vi "Doe_Julabo_Control_subVI.vi"(0 "Julabo CF41 VISA":refnum<visa-resource-name>="COM3", 1 "Data Cluster In":T1={"Current DoE"=[], "SSI 1 Flow Rate"=0.0, "SSI 2 Flow Rate"=0.0, "FLOM 1 Flow Rate"=0.0, "FLOM 2 Flow Rate"=0.0, "Pumps Running?"=FALSE, "Boolean 2"=FALSE, "Boolean 3"=FALSE, "Boolean 4"=FALSE, "At Equilibrium?"=FALSE, "Script Running?"=FALSE, "Current Script Iteration"=0.0, "Total Script Iterations"=0.0, "FLOM Pumps VISA"="COM2", "SSI 1 Pump VISA"="COM76", "SSI 2 Pump VISA"="COM74", "Huber Unistat VISA"="COM1", "SSI 3 Pump VISA"="COM76", "SSI 4 Pump VISA"="COM76", "SSI 4 Flow Rate"=0.0, "SSI 3 Flow Rate"=0.0, "Flow Meter 1 Rate "=0.0, "Flow Meter 2 Rate"=0.0, "Flow Meter 3 Rate"=0.0, "Flow Meter 4 Rate"=0.0, "SSI 1 Flow Setpoint"=0.0, "SSI 2 Flow Setpoint"=0.0, "SSI 3 Flow Setpoint"=0.0, "SSI 4 Flow Setpoint"=0.0, "Temperature Setpoint"=0.0, "Flow meter 3 COM"=17, "Flow meter 5 COM"=18, "Flow meter 4 COM"=19, "Flow meter 2 COM"=16, "Flow meter 1 COM"=15, "Unit"=enum."PSI", "Pressure COM"="COM6", "Julabo Setpoint"=0.0, "Julabo Control"=enum."Internal", "Overtemp"=50.0, "Subtemp"=-20.0, "HeatMax"=50, "CoolMax"=-100, "InternMax"=50.0, "InternMin"=0.0, "Upper Bandlimit"=100.0, "Lower Bandlimit"=0.0, "Julabo CF41 VISA"="COM3", "Xp (0.6K) Int"=0.6, "Tn (3s) Int"=3, "Tv (0s) Int"=0, "Dynamic (0: aperiodic) Int"=enum."aperiodic", "Xp (0.6K) Ext"=0.6, "Tn (3s) Ext"=3, "Tv (0s) Ext"=0, "XpU (0.6K) Ext"=0.6} {"XpU (0.6K) Ext" min=0.1 max=99.9; "Tv (0s) Ext" max=999; "Tn (3s) Ext" min=3 max=9999; "Xp (0.6K) Ext" min=0.1 max=99.9; "Tv (0s) Int" max=999; "Tn (3s) Int" min=3 max=9999; "Xp (0.6K) Int" min=0.1 max=99.9; "Lower Bandlimit" min=0.0 max=200.0; "Upper Bandlimit" min=0.0 max=200.0; "InternMin" format="%.2f"; "InternMax" format="%.2f"; "CoolMax" min=-100 max=0; "HeatMax" max=100; "Subtemp" format="%.2f"; "Overtemp" format="%.2f"; "Julabo Setpoint" format="%.2f"; "Current DoE" format="%0.3f"}, 2 "Selector":i32, 5 "Serial Configuration":T4={"Baud Rate"=4800, "Parity"=2, "Data Bits"=7, "Stop Bits"=10, "Flow Control"=2} {"Flow Control" items=["None", "XON/XOFF", "RTS/CTS", "XON/XOFF & RTS/CTS", "DTR/DSR", "XON/XOFF & DTR/DSR"]; "Stop Bits" items=["1.0"=10, "1.5"=15, "2.0"=20]; "Data Bits" items=["7"=7, "8"=8]; "Parity" items=["None", "Odd", "Even", "Mark", "Space"]; "Baud Rate" items=["300"=300, "600"=600, "1200"=1200, "2400"=2400, "4800"=4800, "9600"=9600, "19200"=19200]}, 7 "RS485-Address (128: RS232)":u32=128, 9 "ID Query? (T: Yes)":bool=TRUE) -> (4 "Data Cluster Out":T1={"Current DoE"=[], "SSI 1 Flow Rate"=0.0, "SSI 2 Flow Rate"=0.0, "FLOM 1 Flow Rate"=0.0, "FLOM 2 Flow Rate"=0.0, "Pumps Running?"=FALSE, "Boolean 2"=FALSE, "Boolean 3"=FALSE, "Boolean 4"=FALSE, "At Equilibrium?"=FALSE, "Script Running?"=FALSE, "Current Script Iteration"=0.0, "Total Script Iterations"=0.0, "FLOM Pumps VISA"="COM2", "SSI 1 Pump VISA"="COM76", "SSI 2 Pump VISA"="COM74", "Huber Unistat VISA"="COM1", "SSI 3 Pump VISA"="COM76", "SSI 4 Pump VISA"="COM76", "SSI 4 Flow Rate"=0.0, "SSI 3 Flow Rate"=0.0, "Flow Meter 1 Rate "=0.0, "Flow Meter 2 Rate"=0.0, "Flow Meter 3 Rate"=0.0, "Flow Meter 4 Rate"=0.0, "SSI 1 Flow Setpoint"=0.0, "SSI 2 Flow Setpoint"=0.0, "SSI 3 Flow Setpoint"=0.0, "SSI 4 Flow Setpoint"=0.0, "Temperature Setpoint"=0.0, "Flow meter 3 COM"=17, "Flow meter 5 COM"=18, "Flow meter 4 COM"=19, "Flow meter 2 COM"=16, "Flow meter 1 COM"=15, "Unit"=enum."PSI", "Pressure COM"="COM6", "Julabo Setpoint"=0.0, "Julabo Control"=enum."Internal", "Overtemp"=50.0, "Subtemp"=-20.0, "HeatMax"=50, "CoolMax"=-100, "InternMax"=50.0, "InternMin"=0.0, "Upper Bandlimit"=100.0, "Lower Bandlimit"=0.0, "Julabo CF41 VISA"="COM3", "Xp (0.6K) Int"=0.6, "Tn (3s) Int"=3, "Tv (0s) Int"=0, "Dynamic (0: aperiodic) Int"=enum."aperiodic", "Xp (0.6K) Ext"=0.6, "Tn (3s) Ext"=3, "Tv (0s) Ext"=0, "XpU (0.6K) Ext"=0.6} {"XpU (0.6K) Ext" min=0.1 max=99.9; "Tv (0s) Ext" max=999; "Tn (3s) Ext" min=3 max=9999; "Xp (0.6K) Ext" min=0.1 max=99.9; "Tv (0s) Int" max=999; "Tn (3s) Int" min=3 max=9999; "Xp (0.6K) Int" min=0.1 max=99.9; "Lower Bandlimit" min=0.0 max=200.0; "Upper Bandlimit" min=0.0 max=200.0; "InternMin" format="%.2f"; "InternMax" format="%.2f"; "CoolMax" min=-100 max=0; "HeatMax" max=100; "Subtemp" format="%.2f"; "Overtemp" format="%.2f"; "Julabo Setpoint" format="%.2f"; "Current DoE" format="%0.3f"}, 15 "device error out":errorcluster)   [LabVIEW 2015, in "JULABO DeviceDriver.lvlib"]
doc: "Advanced event triggered example"
uses:
  <instrlib>/JULABO DeviceDriver/JULABO DeviceDriver.lvlib
  <instrlib>/JULABO DeviceDriver/Examples/Julabo Serial Control.ctl
  --Controls and TypeDefs--/DoE_Control_Cluster.ctl
panel:
  in  "Xp (0.6K) 2":dbl=0.6 min=0.1 max=99.9
  in  "Tn (3s) 2":u16=3 min=3 max=9999
  in  "Tv (0s) 2":u16 max=999
  in  "XpU (0.6K)":dbl=0.6 min=0.1 max=99.9
  in  "Xp (0.6K)":dbl=0.6 min=0.1 max=99.9
  in  "Tn (3s)":u16=3 min=3 max=9999
  in  "Tv (0s)":u16 max=999
  in  "Dynamic (0: aperiodic)":enum16{"aperiodic", "standard"}(ring)
  in  "Control":enum16{"Internal", "External"}(ring)
  out "Internal Temp":dbl format="%.2f"
  out "External Temp":dbl format="%.2f"
  out "Safety Temp":dbl
  out "Excess Temp Protection":dbl
  in  "Setpoint":dbl format="%.2f"
  in  "StartStop":bool
  in  "Upper Bandlimit":dbl=100.0 min=0.0 max=200.0
  in  "Lower Bandlimit":dbl min=0.0 max=200.0
  in  "InternMax":dbl=50.0 format="%.2f"
  in  "InternMin":dbl format="%.2f"
  in  "HeatMax":u8=50 max=100
  in  "CoolMax":i8=-100 min=-100 max=0
  in  "Overtemp":dbl=50.0 format="%.2f"
  in  "Subtemp":dbl=-20.0 format="%.2f"
  out "error out 2":errorcluster caption="error out"
  out "error out":errorcluster
  in  "Registerkartenelement":T2(tab)
  out "Power":i8(slide) scale=-100.0..100.0
  out "Diagram":T3(graph)
  in  "Stopp":bool
  in  "Reset / Default (T: Both)":bool=TRUE
  # "Note: Julabo must be set to Set Temp - RS232\nfor commands to properly write to unit!!!!!"
  # "1. Select the COM-Port and adjust the serial\nconfiguration for your instrument\n2. Adjust the Read cycle\n3. Start the VI by pressing the \"Start\" -Button\n( Arrow button on the top-left corner)\n4. To stop the execution press the \"Stop\" button"
  # "Julabo"
  # "Limits"
  # "PID Control Parameters"
  # "Julabo"
  # "Limits"
  # "PID Control Parameters"
  # "Internal parameters"
  # "External parameters"
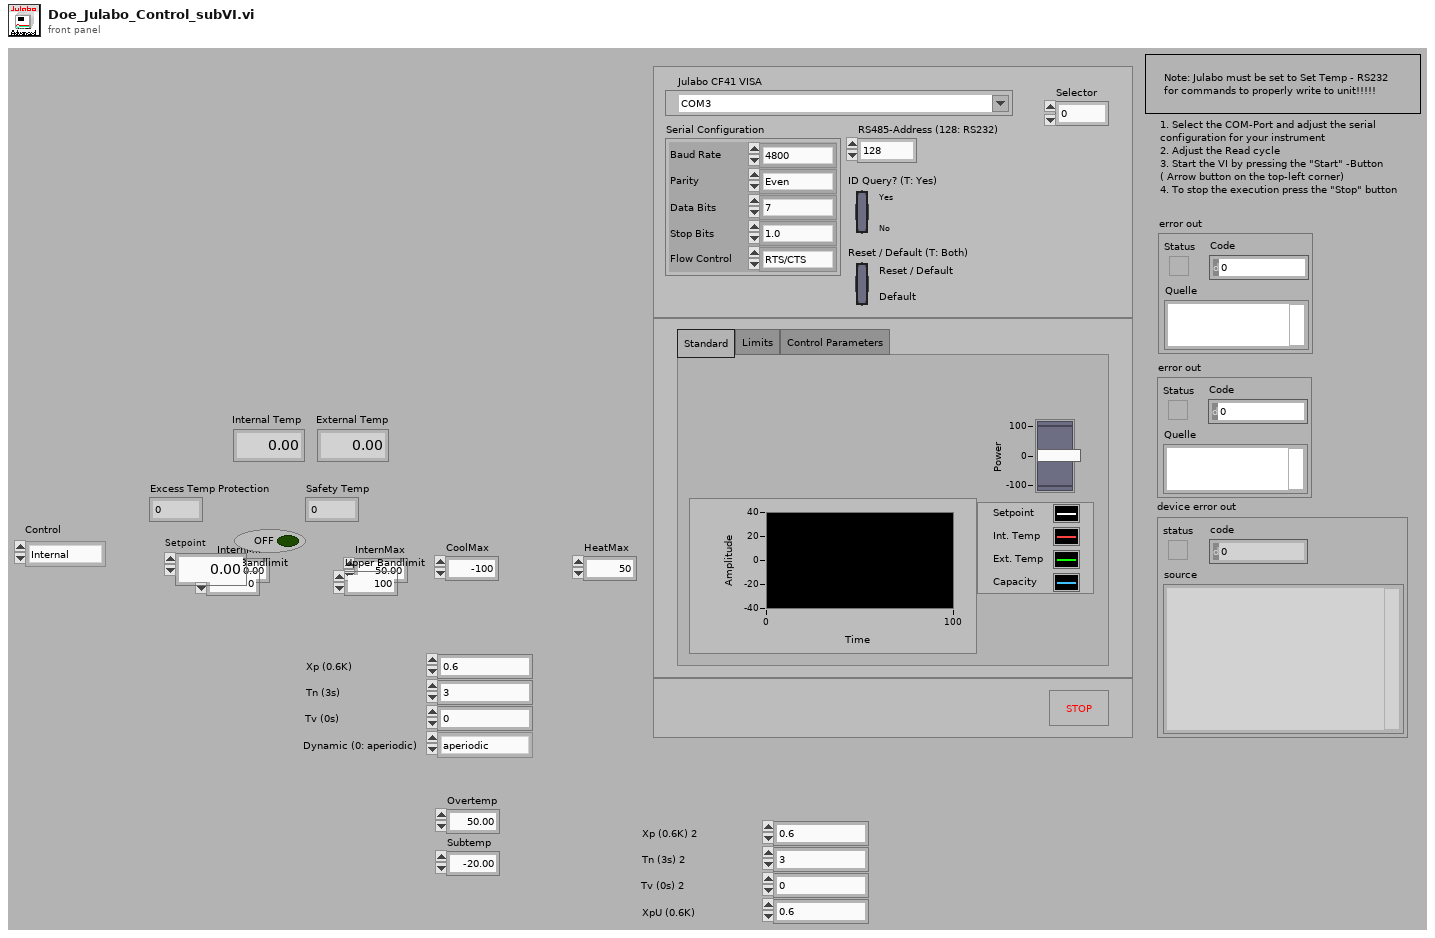
[diagram p1: front panel]
types:
  T1 = typedef "DoE_Control_Cluster.ctl" = cluster{"Current DoE":dbl[][], "SSI 1 Flow Rate":dbl, "SSI 2 Flow Rate":dbl, "FLOM 1 Flow Rate":dbl, "FLOM 2 Flow Rate":dbl, "Pumps Running?":bool, "Boolean 2":bool, "Boolean 3":bool, "Boolean 4":bool, "At Equilibrium?":bool, "Script Running?":bool, "Current Script Iteration":dbl, "Total Script Iterations":dbl, "FLOM Pumps VISA":refnum<visa-resource-name>, "SSI 1 Pump VISA":refnum<visa-resource-name>, "SSI 2 Pump VISA":refnum<visa-resource-name>, "Huber Unistat VISA":refnum<visa-resource-name>, "SSI 3 Pump VISA":refnum<visa-resource-name>, "SSI 4 Pump VISA":refnum<visa-resource-name>, "SSI 4 Flow Rate":dbl, "SSI 3 Flow Rate":dbl, "Flow Meter 1 Rate ":dbl, "Flow Meter 2 Rate":dbl, "Flow Meter 3 Rate":dbl, "Flow Meter 4 Rate":dbl, "SSI 1 Flow Setpoint":dbl, "SSI 2 Flow Setpoint":dbl, "SSI 3 Flow Setpoint":dbl, "SSI 4 Flow Setpoint":dbl, "Temperature Setpoint":dbl, "Flow meter 3 COM":u16, "Flow meter 5 COM":u16, "Flow meter 4 COM":u16, "Flow meter 2 COM":u16, "Flow meter 1 COM":u16, "Unit":enum16{"PSI", "Bar", "cm H2O", "ft H2O", "hectoPascal", "in Hg", "in H2O", "kiloPascal", "milliBar", "mmHg", "MegaPascal", "Numeric Pressure"}, "Pressure COM":refnum<visa-resource-name>, "Julabo Setpoint":dbl, "Julabo Control":enum16{"Internal", "External"}, "Overtemp":dbl, "Subtemp":dbl, "HeatMax":u8, "CoolMax":i8, "InternMax":dbl, "InternMin":dbl, "Upper Bandlimit":dbl, "Lower Bandlimit":dbl, "Julabo CF41 VISA":refnum<visa-resource-name>, "Xp (0.6K) Int":dbl, "Tn (3s) Int":u16, "Tv (0s) Int":u16, "Dynamic (0: aperiodic) Int":enum16{"aperiodic", "standard"}, "Xp (0.6K) Ext":dbl, "Tn (3s) Ext":u16, "Tv (0s) Ext":u16, "XpU (0.6K) Ext":dbl}
  T2 = enum32{"Standard", "Limits", "Control Parameters"}
  T3 = cluster{"Setpoint (out)":dbl, "InternalTemp (out)":dbl, "ExternalTemp (out)":dbl, "Capacity (out)":i8}
  T4 = typedef "Julabo Serial Control.ctl" = cluster{"Baud Rate":u32, "Parity":u16, "Data Bits":u16, "Stop Bits":u16, "Flow Control":u16}
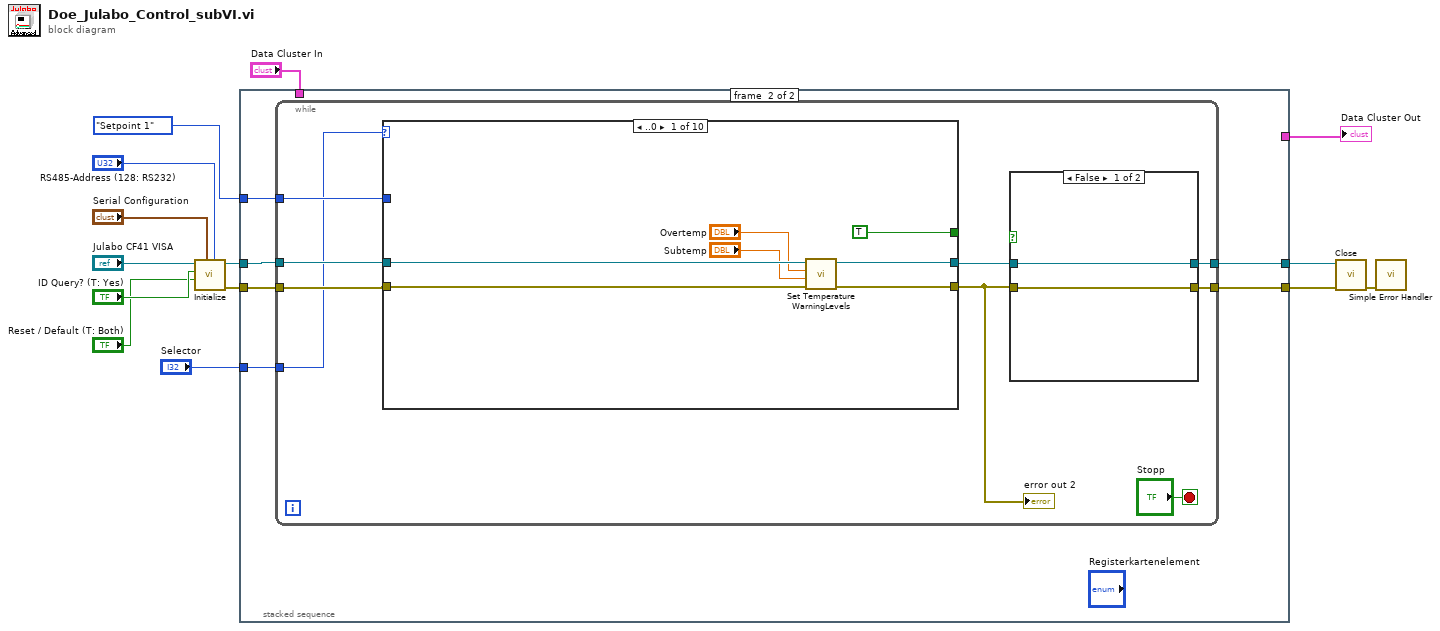
[diagram p0: block diagram]
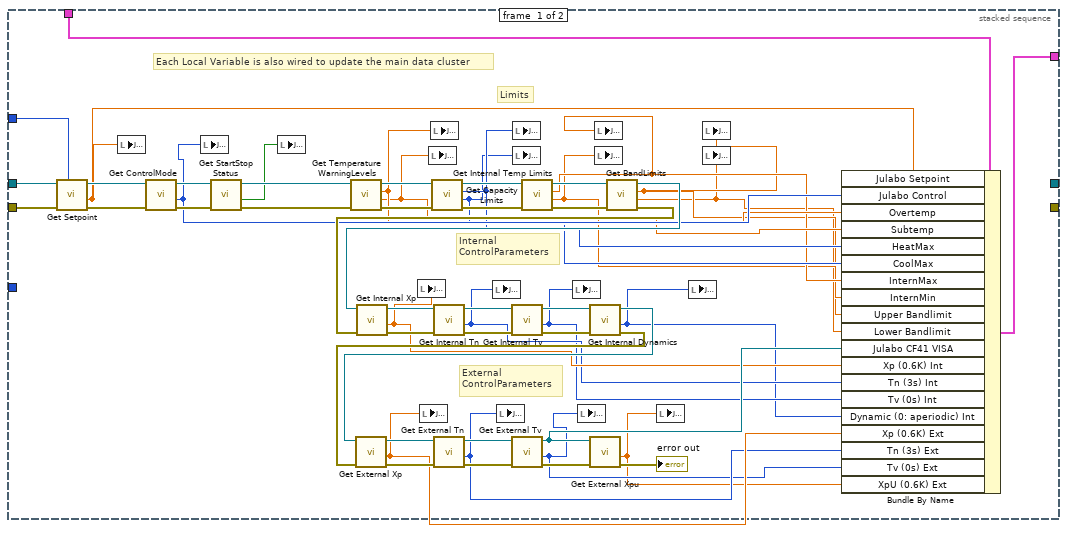
[diagram p2: hidden frame]
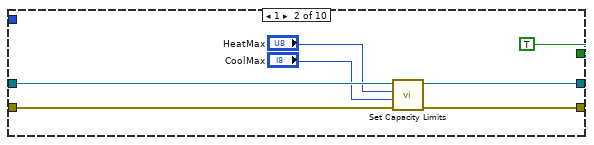
[diagram p3: hidden frame]
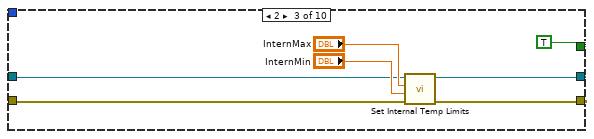
[diagram p4: hidden frame]
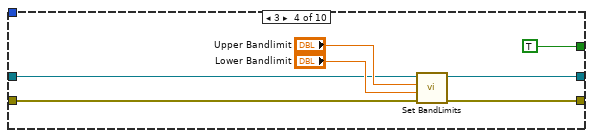
[diagram p5: hidden frame]
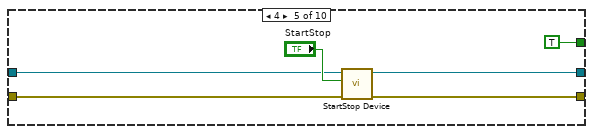
[diagram p6: hidden frame]
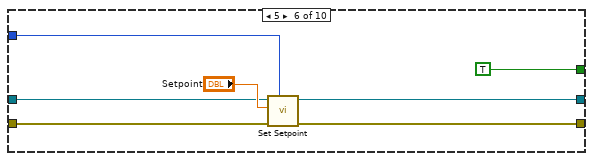
[diagram p7: hidden frame]
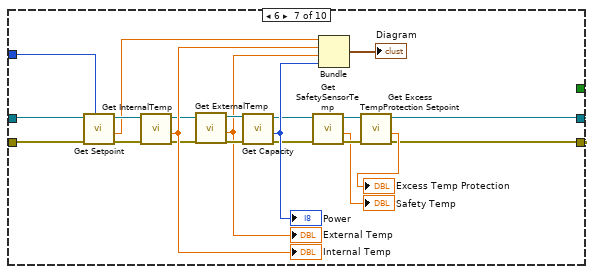
[diagram p8: hidden frame]
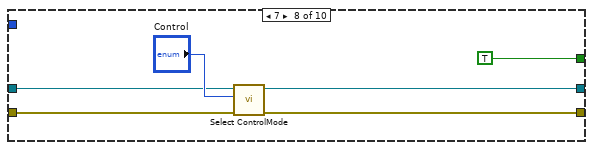
[diagram p9: hidden frame]
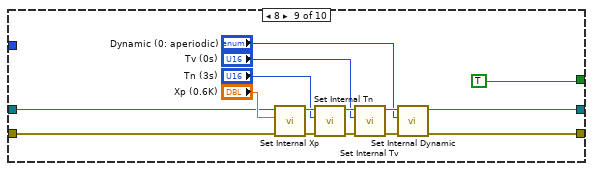
[diagram p10: hidden frame]
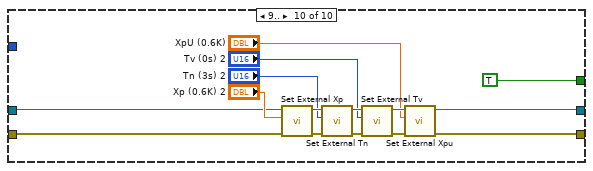
[diagram p11: hidden frame]
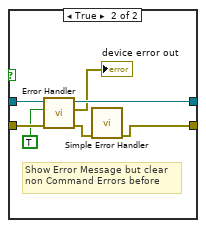
[diagram p12: hidden frame]
diagram:
  n1 = call <instrlib>:"Initialize.vi"("RS485-Address (128: RS232)"="RS485-Address (128: RS232)", "Serial Configuration"="Serial Configuration", "Reset / Default (T: Both)"="Reset / Default (T: Both)", "ID Query? (T: Yes)"="ID Query? (T: Yes)", "VISA resource name"="Julabo CF41 VISA") -> ("error out"=w7:errorcluster, "VISA resource name out"=w8:refnum<visa-resource-name>)  [unwired: 5 in]
  n2 = stacked-sequence {
    tunnel: w8 -> [w40 w69]
    tunnel: w7 -> [w39 w70]
    tunnel: [_ w73] -> w6
    tunnel: [_ w72] -> w5
    tunnel: enum16{"Setpoint 1", "Setpoint 2", "Setpoint 3"}."Setpoint 1" ("Setpointindex") -> [w36 w71]
    tunnel: "Data Cluster In" -> [w35 _]
    tunnel: [w34 _] -> w2
    tunnel: "Selector" -> [_ w68]
    frame #0 {
      # "Each Local Variable is also wired to update the main data cluster"
      # "External\nControlParameters"
      # "Internal\nControlParameters"
      # "Limits"
      n3 = call <instrlib>:"Get Setpoint.vi"("Setpointindex"=w36, "error in (no error)"=w39, "VISA resource name"=w40) -> ("error out"=w37:errorcluster, "Setpoint (out)"=w33:dbl, "VISA resource name out"=w38:refnum<visa-resource-name>)  [unwired: 6 in]
      n4 = local write item#-1(w33) -> ()
      n5 = call <instrlib>:"Get ControlMode.vi"("error in"=w37, "VISA resource name in"=w38) -> ("error out"=w42:errorcluster, "Control (out)"=w32:enum16{"Internal", "External"}, "VISA resource name out"=w46:refnum<visa-resource-name>)  [unwired: 7 in]
      n6 = local write item#-1(w32) -> ()
      n7 = call <instrlib>:"Get StartStop Status.vi"("error in"=w42, "VISA resource name in"=w46) -> ("error out"=w41:errorcluster, "Status"=w43:bool, "VISA resource name out"=w44:refnum<visa-resource-name>)  [unwired: 7 in]
      n8 = local write item#-1(w43) -> ()
      n9 = call <instrlib>:"Get Temperature WarningLevels.vi"("error in (no error)"=w41, "VISA resource name"=w44) -> ("error out"=w64:errorcluster, "Subtemp (out)"=w30:dbl, "Overtemp (out)"=w31:dbl, "VISA resource name out"=w67:refnum<visa-resource-name>)  [unwired: 2 in]
      n10 = local write item#-1(w30) -> ()
      n11 = local write item#-1(w31) -> ()
      n12 = call <instrlib>:"Get Capacity Limits.vi"("error in (no error)"=w64, "VISA resource name"=w67) -> ("error out"=w63:errorcluster, "Maximum cooling capacity(out)"=w28:i8, "Maximum heating capacity(out)"=w29:u8, "VISA resource name out"=w66:refnum<visa-resource-name>)  [unwired: 2 in]
      n13 = local write item#-1(w29) -> ()
      n14 = local write item#-1(w28) -> ()
      n15 = call <instrlib>:"Get Internal Temp Limits.vi"("error in (no error)"=w63, "VISA resource name"=w66) -> ("error out"=w62:errorcluster, "IntMin (out)"=w26:dbl, "IntMax (out)"=w27:dbl, "VISA resource name out"=w65:refnum<visa-resource-name>)  [unwired: 2 in]
      n16 = local write item#-1(w27) -> ()
      n17 = local write item#-1(w26) -> ()
      n18 = call <instrlib>:"Get BandLimits.vi"("error in (no error)"=w62, "VISA resource name"=w65) -> ("error out"=w54:errorcluster, "LowerBand (out)"=w24:dbl, "UpperBand (out)"=w25:dbl, "VISA resource name out"=w55:refnum<visa-resource-name>)  [unwired: 2 in]
      n19 = call <instrlib>:"Get Internal Xp.vi"("error in"=w54, "VISA resource name in"=w55) -> ("error out"=w56:errorcluster, "InternalXp (out)"=w22:dbl, "VISA resource name out"=w57:refnum<visa-resource-name>)  [unwired: 7 in]
      n20 = local write item#-1(w22) -> ()
      n21 = call <instrlib>:"Get Internal Tn.vi"("error in"=w56, "VISA resource name in"=w57) -> ("error out"=w58:errorcluster, "InternalTn (out)"=w21:u16, "VISA resource name out"=w59:refnum<visa-resource-name>)  [unwired: 7 in]
      n22 = local write item#-1(w21) -> ()
      n23 = call <instrlib>:"Get Internal Tv.vi"("error in"=w58, "VISA resource name in"=w59) -> ("error out"=w60:errorcluster, "InternalTv (out)"=w20:u16, "VISA resource name out"=w61:refnum<visa-resource-name>)  [unwired: 7 in]
      n24 = local write item#-1(w20) -> ()
      n25 = call <instrlib>:"Get Internal Dynamics.vi"("error in"=w60, "VISA resource name in"=w61) -> ("error out"=w49:errorcluster, "Dynamic (out)"=w19:enum16{"aperiodic", "standard"}, "VISA resource name out"=w48:refnum<visa-resource-name>)  [unwired: 7 in]
      n26 = call <instrlib>:"Get External Xp.vi"("error in"=w49, "VISA resource name in"=w48) -> ("error out"=w50:errorcluster, "ExternalXp (out)"=w18:dbl, "VISA resource name out"=w47:refnum<visa-resource-name>)  [unwired: 7 in]
      n27 = local write item#-1(w18) -> ()
      n28 = call <instrlib>:"Get External Tn.vi"("error in"=w50, "VISA resource name in"=w47) -> ("error out"=w53:errorcluster, "ExternalTn (out)"=w17:u16, "VISA resource name out"=w52:refnum<visa-resource-name>)  [unwired: 7 in]
      n29 = local write item#-1(w17) -> ()
      n30 = call <instrlib>:"Get External Tv.vi"("error in"=w53, "VISA resource name in"=w52) -> ("error out"=w51:errorcluster, "ExternalTv (out)"=w16:u16, "VISA resource name out"=w23:refnum<visa-resource-name>)  [unwired: 7 in]
      n31 = local write item#-1(w16) -> ()
      n32 = call <instrlib>:"Get External Xpu.vi"("error in"=w51, "VISA resource name in"=w23) -> ("error out"=→"error out":errorcluster, "ExternalXpu (out)"=w15:dbl)  [unwired: 7 in, 1 out]
      n33 = local write item#-1(w15) -> ()
      n34 = local write item#-1(w19) -> ()
      n35 = local write item#-1(w25) -> ()
      n36 = local write item#-1(w24) -> ()
      n37 = Bundle By Name(cluster=w35, "Julabo Setpoint"=w33, "Julabo Control"=w32, "Overtemp"=w31, "Subtemp"=w30, "HeatMax"=w29, "CoolMax"=w28, "InternMax"=w27, "InternMin"=w26, "Upper Bandlimit"=w25, "Lower Bandlimit"=w24, "Julabo CF41 VISA"=w23, "Xp (0.6K) Int"=w22, "Tn (3s) Int"=w21, "Tv (0s) Int"=w20, "Dynamic (0: aperiodic) Int"=w19, "Xp (0.6K) Ext"=w18, "Tn (3s) Ext"=w17, "Tv (0s) Ext"=w16, "XpU (0.6K) Ext"=w15) -> (w34:T1)
    }
    frame #1 {
      n38 = while {
        tunnel: w69 -> [w77]
        tunnel: w70 -> [w78]
        tunnel: [w82] -> w72
        tunnel: [w81] -> w73
        tunnel: w71 -> [w79]
        tunnel: w68 -> [w74]
        stop <- "Stopp" stop-if-true
        n39 = case shown="..0" w74 {
          tunnel: w78 -> [w89 w95 w101 w108 w115 w120 w128 w150 w153 w171]
          tunnel: w77 -> [w88 w96 w100 w107 w114 w121 w127 w149 w152 w170]
          tunnel: [w87 w94 w99 w105 w112 w118 w124 w148 w155 w168] -> w76
          tunnel: [w86 w92 w98 w106 w113 w117 w125 w147 w154 w169] -> w75
          tunnel: [TRUE TRUE TRUE TRUE TRUE TRUE _ TRUE TRUE TRUE] -> _
          tunnel: w79 -> [_ _ _ _ _ w122 w126 _ _ _]
          frame ..0 {
            n40 = call <instrlib>:"Set Temperature WarningLevels.vi"("error in (no error)"=w89, "Subtemp (-20.00°C)"="Subtemp", "Overtemp (50.00°C)"="Overtemp", "VISA resource name"=w88) -> ("error out"=w86:errorcluster, "VISA resource name out"=w87:refnum<visa-resource-name>)  [unwired: 6 in]
          }
          frame 1 {
            n41 = call <instrlib>:"Set Capacity Limits.vi"("error in (no error)"=w95, "Maximum cooling capacity(-100%)"="CoolMax", "Maximum heating capacity(100%)"="HeatMax", "VISA resource name"=w96) -> ("error out"=w92:errorcluster, "VISA resource name out"=w94:refnum<visa-resource-name>)  [unwired: 6 in]
          }
          frame 2 {
            n42 = call <instrlib>:"Set Internal Temp Limits.vi"("error in (no error)"=w101, "InternMin (-20.00 °C)"="InternMin", "InternMax (50.00 °C)"="InternMax", "VISA resource name"=w100) -> ("error out"=w98:errorcluster, "VISA resource name out"=w99:refnum<visa-resource-name>)  [unwired: 6 in]
          }
          frame 3 {
            n43 = call <instrlib>:"Set BandLimits.vi"("error in (no error)"=w108, "Lower Bandlimit (200K)"="Lower Bandlimit", "Upper Bandlimit (200K)"="Upper Bandlimit", "VISA resource name"=w107) -> ("error out"=w106:errorcluster, "VISA resource name out"=w105:refnum<visa-resource-name>)  [unwired: 6 in]
          }
          frame 4 {
            n44 = call <instrlib>:"StartStop Device.vi"("error in (no error)"=w115, "Start/Stop (f:Stop)"="StartStop", "VISA resource name"=w114) -> ("error out"=w113:errorcluster, "VISA resource name out"=w112:refnum<visa-resource-name>)  [unwired: 7 in]
          }
          frame 5 {
            n45 = call <instrlib>:"Set Setpoint.vi"("Setpointindex (Setpoint1: Default)"=w122, "error in (no error)"=w120, "newSetpoint (20.00°C)"="Setpoint", "VISA resource name"=w121) -> ("error out"=w117:errorcluster, "VISA resource name out"=w118:refnum<visa-resource-name>)  [unwired: 6 in]
          }
          frame 6 {
            n46 = call <instrlib>:"Get Setpoint.vi"("Setpointindex"=w126, "error in (no error)"=w128, "VISA resource name"=w127) -> ("error out"=w145:errorcluster, "Setpoint (out)"=w141:dbl, "VISA resource name out"=w144:refnum<visa-resource-name>)  [unwired: 6 in]
            n47 = call <instrlib>:"Get InternalTemp.vi"("error in (no error)"=w145, "VISA resource name"=w144) -> ("error out"=w139:errorcluster, "InternalTemp (out)"=w142:dbl, "VISA resource name out"=w140:refnum<visa-resource-name>)  [unwired: 7 in]
            "Internal Temp" <- w142
            n48 = call <instrlib>:"Get ExternalTemp.vi"("error in (no error)"=w139, "VISA resource name"=w140) -> ("error out"=w137:errorcluster, "ExternalTemp (out)"=w135:dbl, "VISA resource name out"=w138:refnum<visa-resource-name>)  [unwired: 6 in, 1 out]
            "External Temp" <- w135
            n49 = call <instrlib>:"Get Capacity.vi"("error in (no error)"=w137, "VISA resource name"=w138) -> ("error out"=w131:errorcluster, "Capacity (out)"=w136:i8, "VISA resource name out"=w134:refnum<visa-resource-name>)  [unwired: 7 in]
            "Power" <- w136
            n50 = call <instrlib>:"Get SafetySensorTemp.vi"("error in (no error)"=w131, "VISA resource name"=w134) -> ("error out"=w132:errorcluster, "Safetytemp (out)"=→"Safety Temp":dbl, "VISA resource name out"=w133:refnum<visa-resource-name>)  [unwired: 7 in]
            n51 = Bundle("Setpoint (out)"=w141, "InternalTemp (out)"=w142, "ExternalTemp (out)"=w135, "Capacity (out)"=w136) -> (→"Diagram":T3)  [unwired: 1 in]
            n52 = call <instrlib>:"Get Excess TempProtection Setpoint.vi"("error in (no error)"=w132, "VISA resource name"=w133) -> ("error out"=w125:errorcluster, "ExcessTempProtection(out)"=→"Excess Temp Protection":dbl, "VISA resource name out"=w124:refnum<visa-resource-name>)  [unwired: 7 in]
          }
          frame 7 {
            n53 = call <instrlib>:"Select ControlMode.vi"("error in (no error)"=w150, "Control (0: Internal)"="Control", "VISA resource name"=w149) -> ("error out"=w147:errorcluster, "VISA resource name out"=w148:refnum<visa-resource-name>)  [unwired: 7 in]
          }
          frame 8 {
            n54 = call <instrlib>:"Set Internal Xp.vi"("error in (no error)"=w153, "Xp (0.6K)"="Xp (0.6K)", "VISA resource name"=w152) -> ("error out"=w164:errorcluster, "VISA resource name out"=w163:refnum<visa-resource-name>)  [unwired: 7 in]
            n55 = call <instrlib>:"Set Internal Tn.vi"("error in (no error)"=w164, "Tn (3s)"="Tn (3s)", "VISA resource name"=w163) -> ("error out"=w166:errorcluster, "VISA resource name out"=w165:refnum<visa-resource-name>)  [unwired: 7 in]
            n56 = call <instrlib>:"Set Internal Tv.vi"("error in (no error)"=w166, "Tv (0s)"="Tv (0s)", "VISA resource name"=w165) -> ("error out"=w158:errorcluster, "VISA resource name out"=w159:refnum<visa-resource-name>)  [unwired: 7 in]
            n57 = call <instrlib>:"Set Internal Dynamic.vi"("error in (no error)"=w158, "Dynamic (0: aperiodic)"="Dynamic (0: aperiodic)", "VISA resource name"=w159) -> ("error out"=w154:errorcluster, "VISA resource name out"=w155:refnum<visa-resource-name>)  [unwired: 7 in]
          }
          frame 9.. {
            n58 = call <instrlib>:"Set External Xp.vi"("error in (no error)"=w171, "Xp (0.6K)"="Xp (0.6K) 2", "VISA resource name"=w170) -> ("error out"=w179:errorcluster, "VISA resource name out"=w178:refnum<visa-resource-name>)  [unwired: 7 in]
            n59 = call <instrlib>:"Set External Tn.vi"("error in (no error)"=w179, "Tn (3s)"="Tn (3s) 2", "VISA resource name"=w178) -> ("error out"=w181:errorcluster, "VISA resource name out"=w180:refnum<visa-resource-name>)  [unwired: 7 in]
            n60 = call <instrlib>:"Set External Tv.vi"("error in (no error)"=w181, "Tv (0s)"="Tv (0s) 2", "VISA resource name"=w180) -> ("error out"=w173:errorcluster, "VISA resource name out"=w174:refnum<visa-resource-name>)  [unwired: 7 in]
            n61 = call <instrlib>:"Set External Xpu.vi"("error in (no error)"=w173, "XpU (0.6K)"="XpU (0.6K)", "VISA resource name"=w174) -> ("error out"=w169:errorcluster, "VISA resource name out"=w168:refnum<visa-resource-name>)  [unwired: 7 in]
          }
        }
        "error out 2" <- w75
        n62 = case shown="False" {
          selector: _ -> [_ _]
          tunnel: w76 -> [w183 w188]
          tunnel: [w183 w186] -> w82
          tunnel: w75 -> [w182 w189]
          tunnel: [w182 w190] -> w81
          frame False {
          }
          frame True {
            # "Show Error Message but clear\nnon Command Errors before"
            n63 = call <instrlib>:"Error Handler.vi"("error in (no error)"=w189, "ClearDeviceError (false)"=TRUE, "VISA resource name"=w188) -> ("error out"=w187:errorcluster, "device error out"=→"device error out":errorcluster, "VISA resource name out"=w186:refnum<visa-resource-name>)  [unwired: 5 in, 1 out]
            n64 = call <vilib>:"Simple Error Handler.vi"("error in (no error)"=w187) -> ("error out"=w190:errorcluster)  [unwired: 4 in, 4 out]
          }
        }
      }
    }
  }
  "Data Cluster Out" <- w2
  n65 = call <instrlib>:"Close.vi"("error in (no error)"=w6, "VISA resource name"=w5) -> ("error out"=w12:errorcluster)  [unwired: 9 in]
  n66 = call <vilib>:"Simple Error Handler.vi"("error in (no error)"=w12) -> ()  [unwired: 4 in, 5 out]
